vi "SendMsgBack.vi"(0 "reference in":refnum<class "Proccess.lvclass">, 5 "message in":T1, 7 "name":string, 9 "value":string, 11 "error in (no error)":errorcluster) -> (4 "reference out":refnum<class "Proccess.lvclass">, 15 "error out":errorcluster)   [LabVIEW 2019, in "Proccess.lvclass"]
uses:
  Proccess_class/Proccess.lvclass
  MessageInterface_class/Message.ctl
  Proccess_class/Proccess.lvclass/Proccess.ctl
  MessageInterface_class/MessageInterface.lvclass
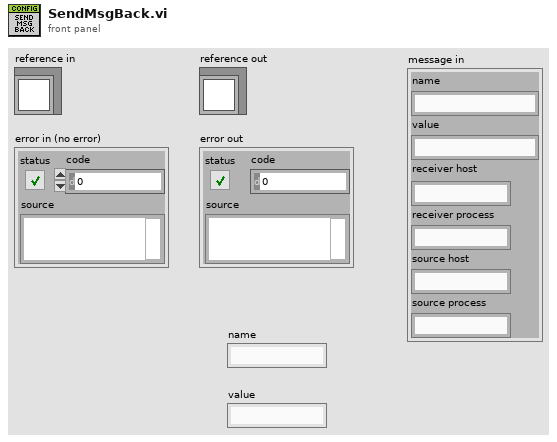
[diagram p1: front panel]
types:
  T1 = typedef "MessageInterface.lvclass/Message.ctl" = cluster{"name":string, "value":string, "receiver host":string, "receiver process":string, "source host":string, "source process":string}
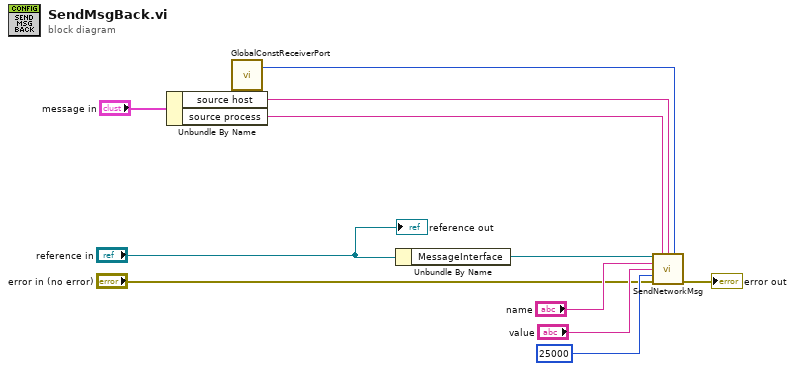
[diagram p0: block diagram]
diagram:
  n1 = Unbundle By Name("message in") -> ("source host"=w9:string, "source process"=w8:string)
  n2 = call "GlobalConstReceiverPort.vi"() -> ("receiver port (0)"=w1:u16)  [unwired: 3 in]
  n3 = Unbundle By Name("reference in") -> ("MessageInterface"=w11:refnum<class "MessageInterface.lvclass">)
  n4 = call-dynamic "SendNetworkMsg.vi"("reference in"=w11, "receiver process"=w8, "receiver host"=w9, "receiver port (0)"=w1, "name"="name", "value"="value", "timeout (25000 ms)"=25000, "error in (no error)"="error in (no error)") -> ("error out"=→"error out":errorcluster)  [unwired: 5 in, 2 out]
  "reference out" <- "reference in"
